vi "Pockels Cal-Obtain power meter AI string.vi"() -> (1 "DAQmx Chan.Power meter AI":tag, 3 "Power meter AI (string)":string)   [LabVIEW 2013]
uses:
  Typedefs/HW config states enum.ctl
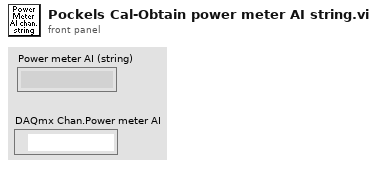
[diagram p1: front panel]
types:
  T1 = typedef "HW config states enum.ctl" = enum16{"Load from file", "Save to file", "Write all", "Read all", "Write XY stage settings", "Write DAQ FPGA settings", "Write Control FPGA settings", "Write Phys Channels", "Clear", "Compare from file"}
  T2 = typedef "Sys Configuration.ctl" = cluster{"XY Stage":T3, "DAQ FPGA":T4, "Control system":T8, "Encoder":T9, "DAQmx Chan":T10, "Computer MAC address":string, "Cam VidRec":T11, "Externalise Triggers":bool, "Laser wavelength (nm)":dbl}
  T3 = typedef "XY Stage config cluster.ctl" = cluster{"COM port":refnum<visa-resource-name>, "XY stage available":bool}
  T4 = typedef "DAQ FPGA config cluster.ctl" = cluster{"Ref":T5, "Target":T6, "Clock Freq (MHz) ":dbl, "input card type":T7, "Samples Wait after Trigger":u16, "AOD fill":u16, "StartupDelay":i32, "Slip Cycle (clock cycles)":u32, "Add Cycle":bool}
  T5 = typedef "FPGA Ref.ctl" = refnum<k20>
  T6 = typedef "nirio_resource_hc.ctl" = tag
  T7 = typedef "FPGA input type AC-DC.ctl" = enum16{"AC Card", "DC Card"}
  T8 = typedef "CTRL system config cluster.ctl" = cluster{"Ethernet opened":bool, "Ethernet Port":u32, "Ctrl FPGA available":bool, "Ctrl FPGA Clock (MHz)":dbl, "Ctrl system MAC address":string, "Control system.Network adapter name":string, "AOD 1 Amplitude":i16, "AOD 2 Amplitude":i16, "AOD 3 Amplitude":i16, "AOD 4 Amplitude":i16, "Data Time Interval (ns)":dbl, "T0 (ns)":dbl, "Ta (ns)":dbl}
  T9 = typedef "Encoder config cluster.ctl" = cluster{"IP address":string, "Port":u16, "Encoder available":bool, "Wheel radius (cm)":dbl}
  T10 = typedef "DAQmx physical channels cluster.ctl" = cluster{"Pockels AO":tag, "Hard shutter AO":tag, "PMT AOs":tag, "Power meter AI":tag}
  T11 = typedef "Cam VidRec HW config setup cluster.ctl" = cluster{"DO flag-Video record":tag, "DO flag-Trial start":tag, "VidRec available":bool}
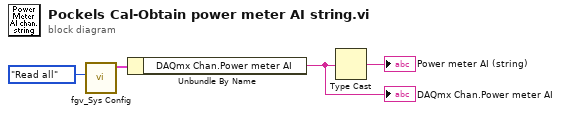
[diagram p0: block diagram]
diagram:
  n1 = call "fgv_Sys Config.vi"("Function"=HW_config_states_enum."Read all") -> ("System Config out"=w3:T2)  [unwired: 9 in, 1 out]
  n2 = Unbundle By Name(w3) -> ("DAQmx Chan.Power meter AI"=w1:tag)
  "DAQmx Chan.Power meter AI" <- w1
  n3 = Type Cast(x=w1) -> (*(type *) &x=→"Power meter AI (string)":string)  [unwired: 1 in]
